vi "grSim Command.vi"(8 "FIRASim?":bool=TRUE, 9 "Robots":T1[](array[typedef]), 10 "isteamyellow":bool=TRUE, 11 "timestamp":dbl format="%#_13g") -> (1 "Command":u8[](array[numeric]))   [LabVIEW 2018]
uses:
  Convert AI Robot to Robot Command Folder/grSim/grSim Robot Command.ctl
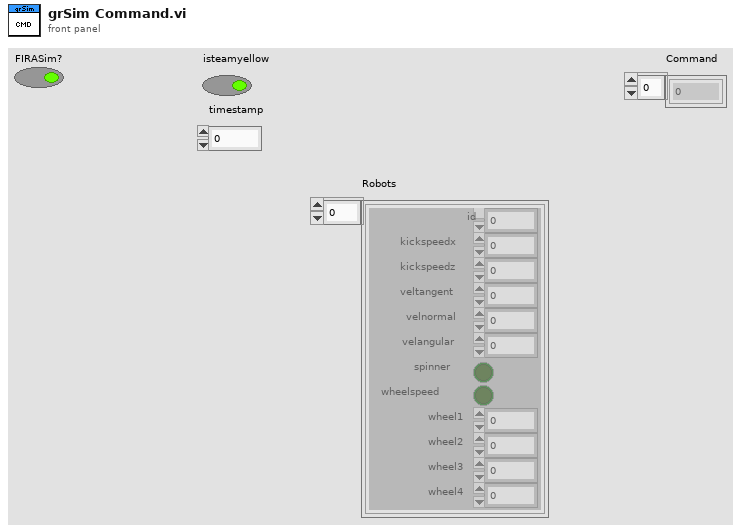
[diagram p1: front panel]
types:
  T1 = typedef "grSim Robot Command.ctl" = cluster{"id":u32, "kickspeedx":sgl, "kickspeedz":sgl, "veltangent":sgl, "velnormal":sgl, "velangular":sgl, "spinner":bool, "wheelspeed":bool, "wheel1":sgl, "wheel2":sgl, "wheel3":sgl, "wheel4":sgl}
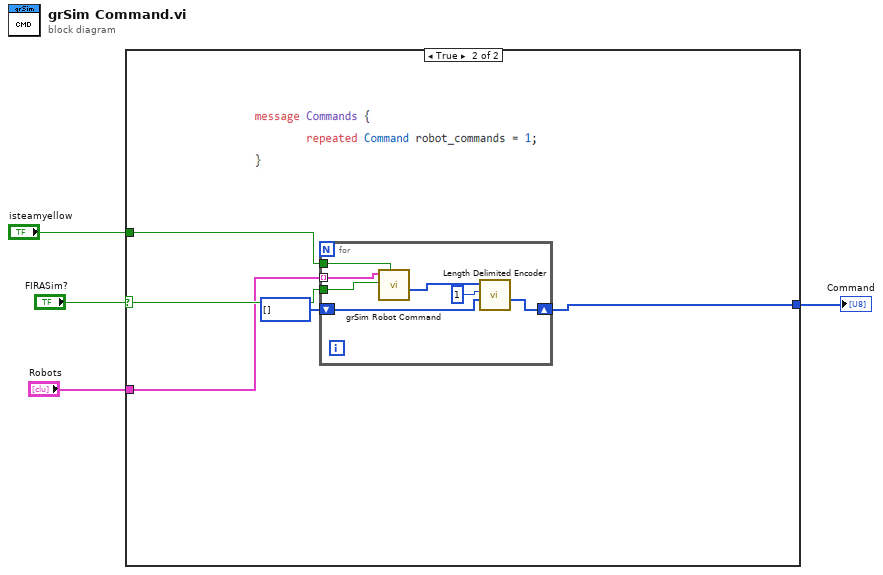
[diagram p0: block diagram]
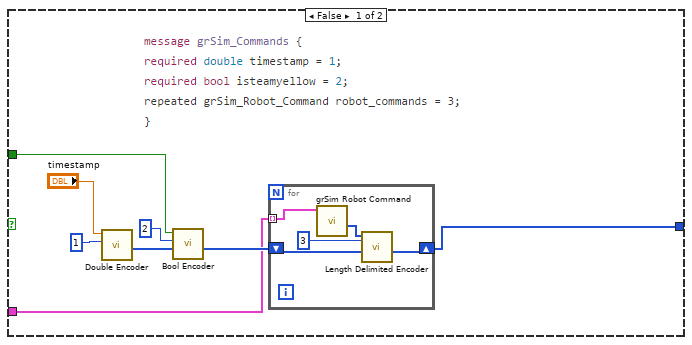
[diagram p2: hidden frame]
diagram:
  n1 = case shown="True" "FIRASim?" {
    selector: "FIRASim?" -> [_ w21]
    tunnel: "isteamyellow" -> [w7 w20]
    tunnel: "Robots" -> [w6 w19]
    tunnel: [w5 w22] -> w1
    frame False {
      n2 = call "Double Encoder.vi"("Key"=u32 1, "Value"="timestamp") -> ("Array"=w11:u8[])  [unwired: 9 in]
      n3 = call "Bool Encoder.vi"("Array In"=w11, "Key"=u32 2, "Value"=w7) -> ("Array"=w8:u8[])  [unwired: 8 in]
      n4 = for {
        shift-right: [w14] -> w5
        shift-left: w8 -> [w15]
        tunnel: w6 -> [w17] mode=indexing
        n5 = call "grSim Robot Command.vi"("Robots"=w17) -> ("Array"=w16:u8[])  [unwired: 10 in]
        n6 = call "Length Delimited Encoder.vi"("Array In"=w15, "Key"=u32 3, "Array In 2"=w16) -> ("Array"=w14:u8[])  [unwired: 8 in]
      }
    }
    frame True {
      n7 = for {
        tunnel: w20 -> [w28]
        shift-right: [w29] -> w22
        shift-left: u8[] [] ("Array") -> [w24]
        tunnel: w19 -> [w25] mode=indexing
        tunnel: w21 -> [w23]
        n8 = call "grSim Robot Command.vi"("YellowTeam?"=w28, "FIRASim?"=w23, "Robots"=w25) -> ("Array"=w26:u8[])  [unwired: 8 in]
        n9 = call "Length Delimited Encoder.vi"("Array In"=w24, "Key"=u32 1, "Array In 2"=w26) -> ("Array"=w29:u8[])  [unwired: 8 in]
      }
    }
  }
  "Command" <- w1
